vi "Solve1.vi"(8 "Error In":errorcluster, 11 "object in":refnum<class "2024_16.lvclass">) -> (0 "Error Out":errorcluster, 2 "Result":u64, 3 "object out":refnum<class "2024_16.lvclass">)   [LabVIEW 2023, in "2024_16.lvclass"]
uses:
  2024_16.lvclass
  2024_16.lvclass/2024_16.ctl
  Common/AOC_Direction.ctl
  Common/AOC_XY(I32).ctl
  Common/AOC_XY.ctl
panel:
  out "Array":T1(array[cluster])
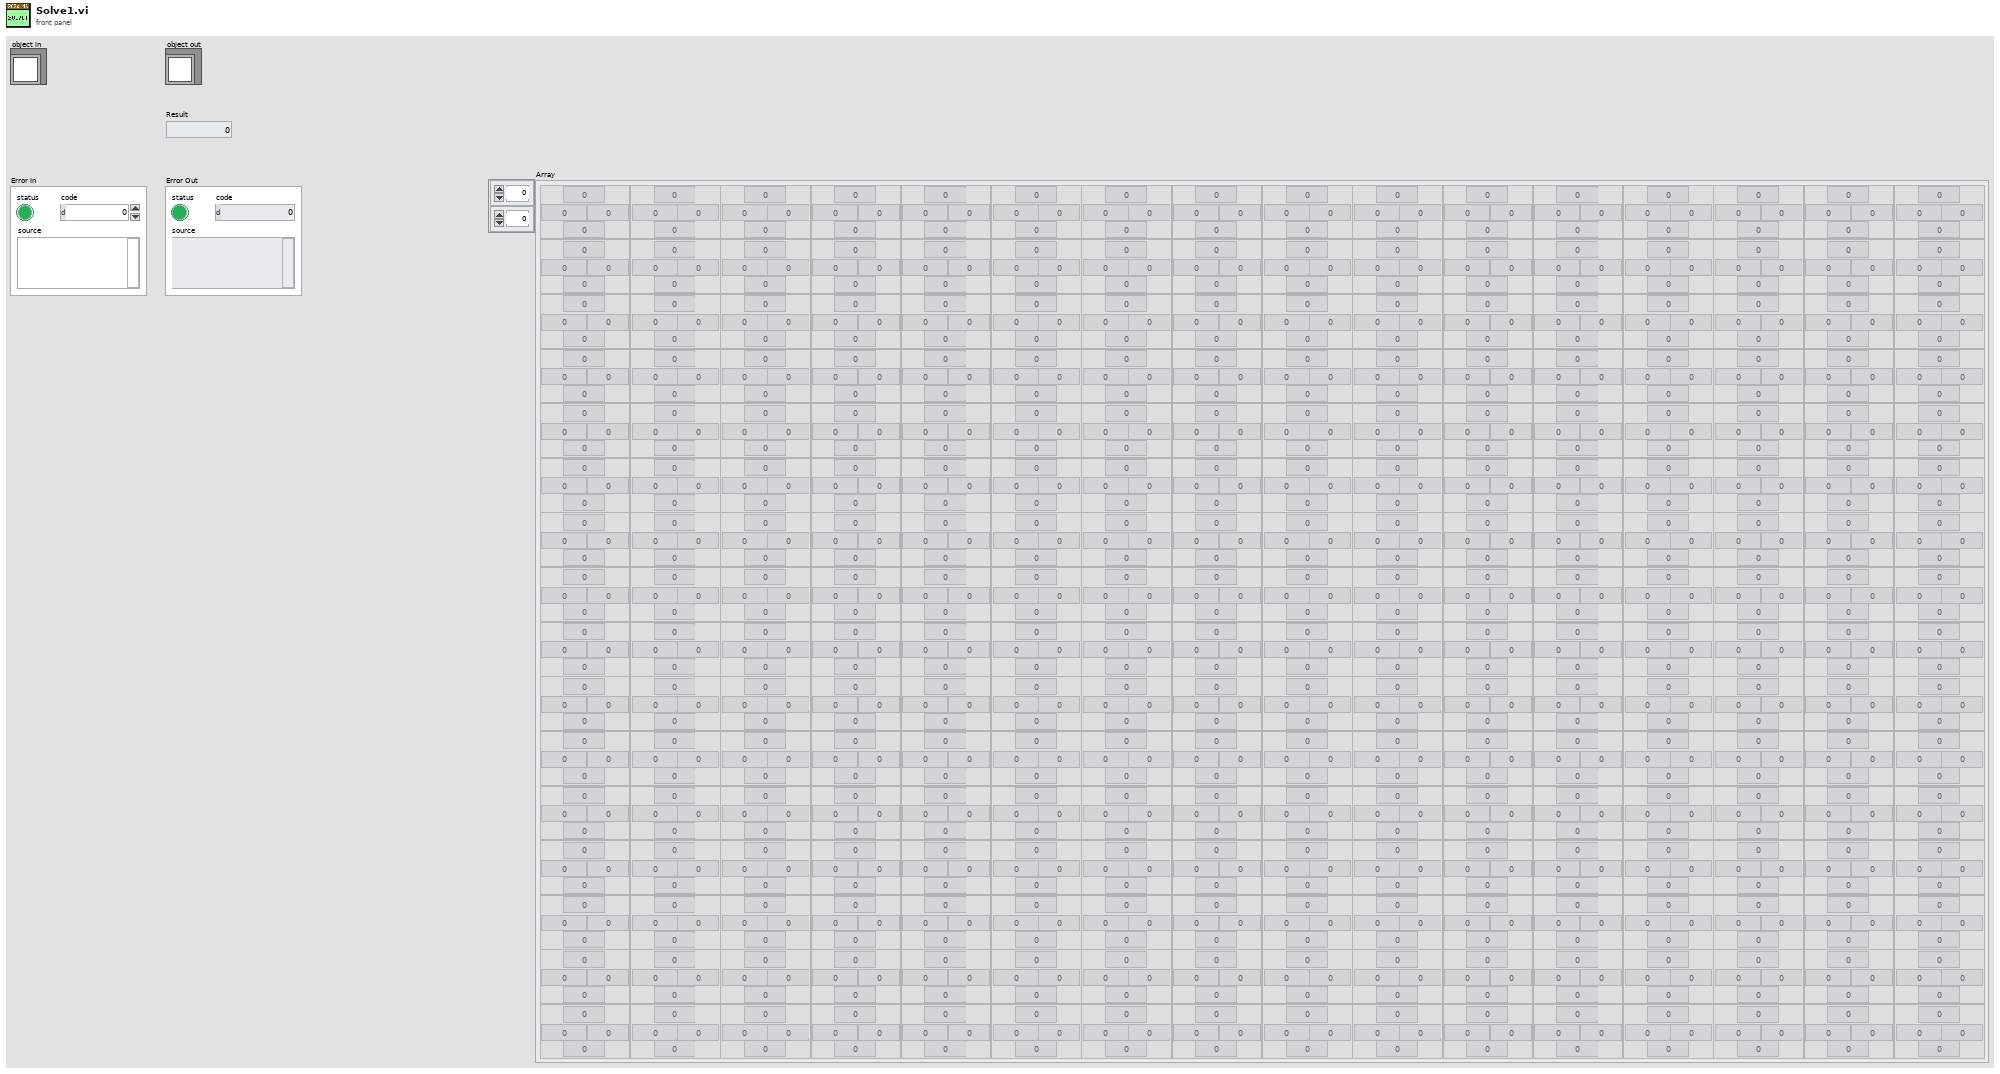
[diagram p1: front panel]
types:
  T1 = cluster{"Up":i32, "Right":i32, "Down":i32, "Left":i32}[][]
  T2 = cluster{"Up":u64, "Right":u64, "Down":u64, "Left":u64}
  T3 = typedef "AOC_Direction.ctl" = enum16{"Up", "Right", "Down", "Left"}
  T4 = typedef "AOC_XY(I32).ctl" = cluster{"X":i32, "Y":i32}
  T5 = map{T4, cluster{"Up":u64, "Right":u64, "Down":u64, "Left":u64}}
  T6 = typedef "AOC_XY.ctl" = cluster{"X":u64, "Y":u64}
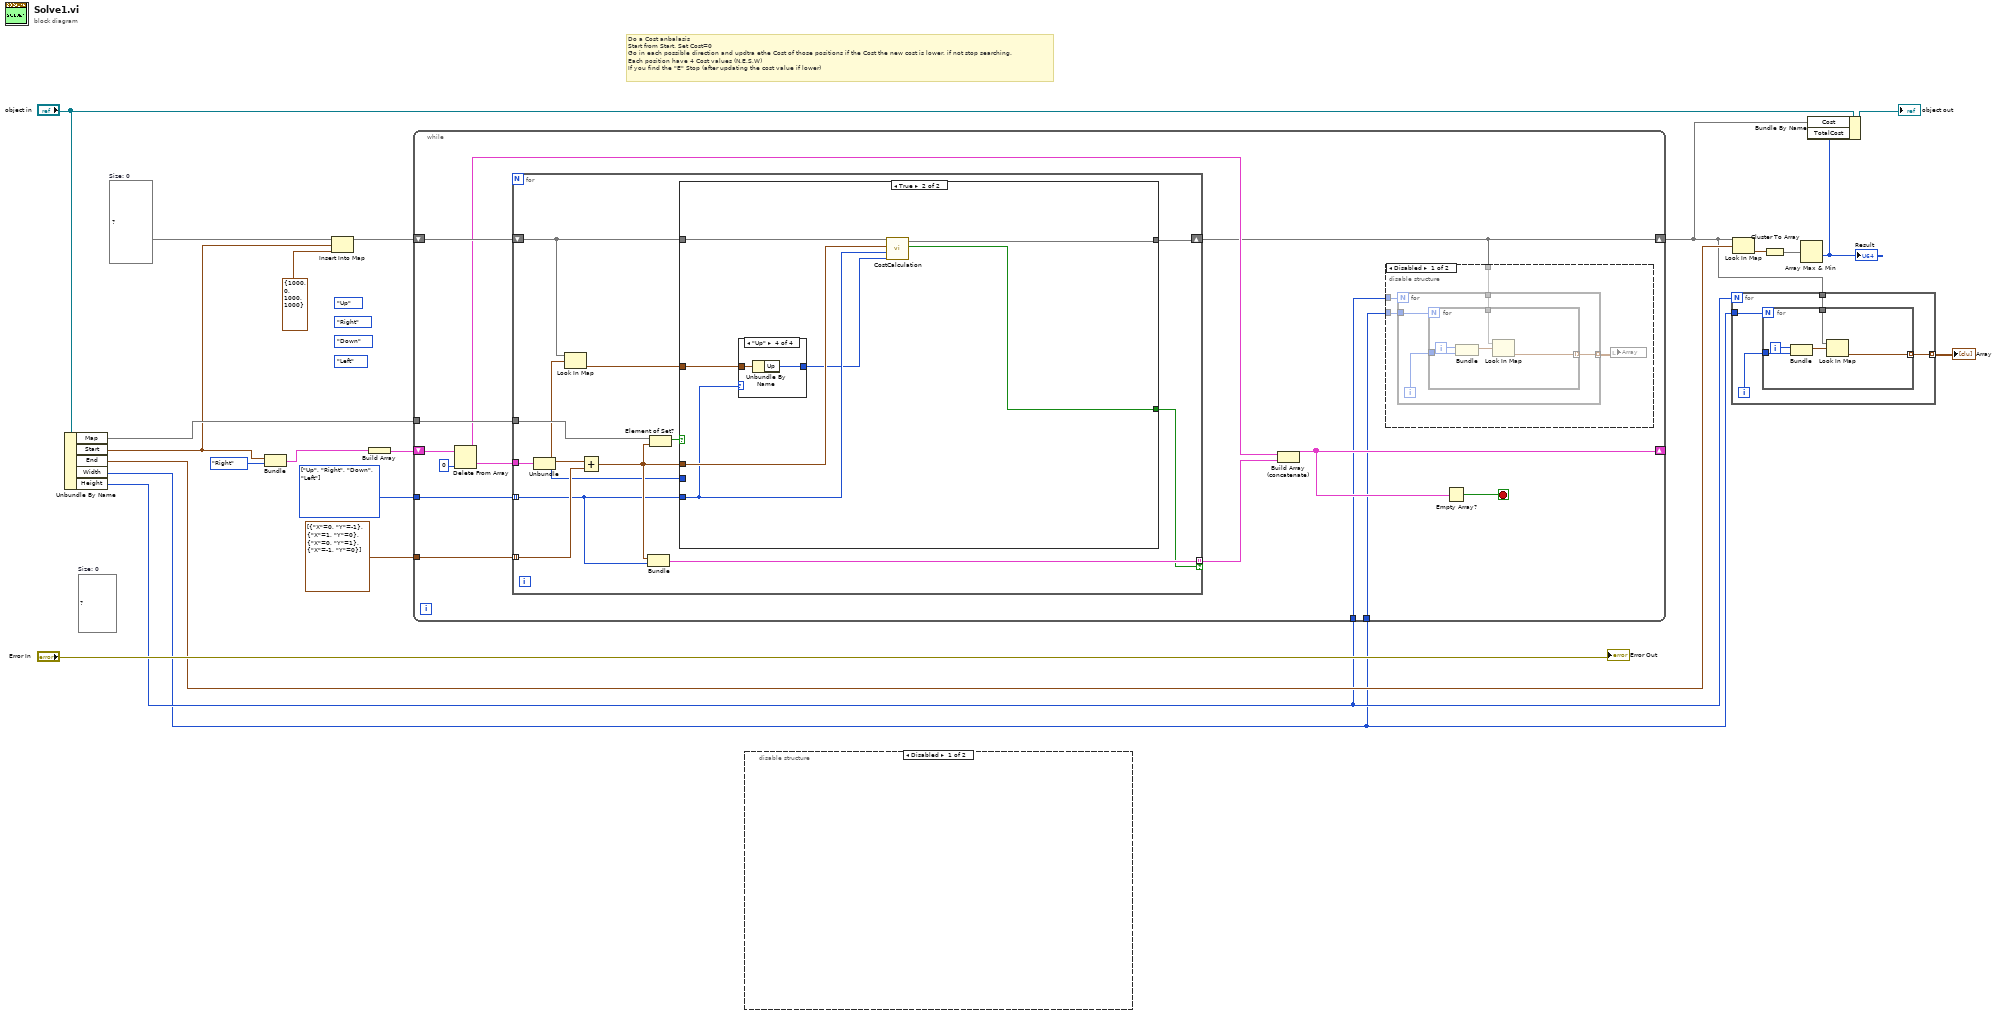
[diagram p0: block diagram]
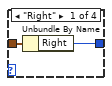
[diagram p5: hidden frame]
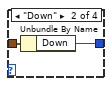
[diagram p6: hidden frame]
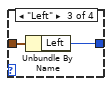
[diagram p7: hidden frame]
diagram:
  (unwired) AOC_Direction."Left" ("Enum")
  (unwired) AOC_Direction."Down" ("Enum")
  (unwired) AOC_Direction."Right" ("Enum")
  (unwired) AOC_Direction."Up" ("Enum")
  w16 = T3[] [enum."Up", enum."Right", enum."Down", enum."Left"] items=["Up", "Right", "Down", "Left"]
  w18 = T5 {}  # Size: 0
  (unwired) map{T6, i32} {}  # Size: 0
  # "Do a Cost anbalasis\nStart from Start. Set Cost=0\nGo in each possible direction and updtra ethe Cost of those positions if the Cost the new cost is lower, if not stop searching.\nEach position have 4 Cost values (N,E,S,W)\nIf you find the \"E\" Stop (after updating the cost value if lower)"
  n1 = Unbundle By Name("object in") -> ("Map"=w14:set{T4}, "Start"=w12:T4, "End"=w9:T4, "Width"=w2:i32, "Height"=w3:i32)
  n2 = Bundle("Start"=w12, AOC_Direction."Right") -> (w11:cluster{"Start":T4, T3})  [unwired: 1 in]
  n3 = Insert Into Map(map in=w18, key=w12, value=T2 {"Up"=1000, "Right"=0, "Down"=1000, "Left"=1000} ("input cluster")) -> (map out=w17:T5)  [unwired: 2 out]
  n4 = Build Array(w11) -> (w19:cluster{"Start":T4, T3}[])
  n5 = while {
    shift-right: [w26] -> _
    shift-left: w19 -> [w35]
    shift-right: [w23] -> w4
    shift-left: w17 -> [w30]
    tunnel: w16 -> [w33]
    tunnel: cluster{"X":i32, "Y":i32}[] [{"X"=0, "Y"=-1}, {"X"=1, "Y"=0}, {"X"=0, "Y"=1}, {"X"=-1, "Y"=0}] ("Array") -> [w32]
    tunnel: w14 -> [w31]
    tunnel: w2 -> [w25]
    tunnel: w3 -> [w24]
    stop <- w22 stop-if-true
    n6 = Delete From Array(array=w35, index=0) -> (deleted portion=w34:cluster{"Start":T4, T3}, array with subset deleted=w29:cluster{"Start":T4, T3}[])  [unwired: 1 in]
    n7 = for {
      tunnel: w34 -> [w59]
      tunnel: w33 -> [w50] mode=indexing
      tunnel: w32 -> [w61] mode=indexing
      tunnel: w31 -> [w60]
      shift-right: [w58] -> w23
      shift-left: w30 -> [w53]
      tunnel: [w54] -> w27 mode=indexing if=w49
      n8 = Unbundle(w59) -> ("Start"=w52:T4, w55:T3)
      n9 = Look In Map(map=w53, key=w52) -> (value=w51:T2)  [unwired: 1 in, 1 out]
      n10 = Add(x=w52, y=w61) -> (x+y=w56:T4)
      n11 = Bundle("Start"=w56, "Enum"=w50) -> (w54:cluster{"Start":T4, "Enum":T3})  [unwired: 1 in]
      n12 = Element of Set?(10:w56, 11:w60) -> (3:w57:bool)
      n13 = case shown="True" w57 {
        tunnel: w55 -> [_ _]
        tunnel: w50 -> [_ w64]
        tunnel: w53 -> [w62 w69]
        tunnel: [w62 w68] -> w58
        tunnel: w56 -> [_ w66]
        tunnel: w51 -> [_ w65]
        tunnel: [_ w67] -> w49
        frame False {
        }
        frame True {
          n14 = case shown="\"Up\"" w64 {
            tunnel: w65 -> [w71 w73 w75 w77]
            tunnel: [w70 w72 w74 w76] -> w63
            frame "Right" {
              n15 = Unbundle By Name(w71) -> ("Right"=w70:u64)
            }
            frame "Down" {
              n16 = Unbundle By Name(w73) -> ("Down"=w72:u64)
            }
            frame "Left" {
              n17 = Unbundle By Name(w75) -> ("Left"=w74:u64)
            }
            frame "Up" {
              n18 = Unbundle By Name(w77) -> ("Up"=w76:u64)
            }
          }
          n19 = call "CostCalculation.vi"("PrevisouCost"=w63, "Direction"=w64, "Position"=w66, "CostIn"=w69) -> ("CostLower"=w67:bool, "CostOut"=w68:T5)  [unwired: 4 in, 2 out]
        }
      }
    }
    n20 = Build Array (concatenate)(w29, w27) -> (w26:cluster{"Start":T4, "Enum":T3}[])
    n21 = disable-structure shown="Disabled" {
      disable-tunnel: w25 -> [w39 _]
      disable-tunnel: w24 -> [w38 _]
      disable-tunnel: w23 -> [w37 _]
      frame Disabled {
        n22 = for {
          N: w38 -> [_]
          tunnel: w39 -> [w43]
          tunnel: w37 -> [w41]
          tunnel: [w40] -> w36 mode=indexing
          i -> [w42]
          n23 = for {
            N: w43 -> [_]
            tunnel: w42 -> [w47]
            tunnel: w41 -> [w46]
            tunnel: [w44] -> w40 mode=indexing
            i -> [w48]
            n24 = Bundle(w48, w47) -> (w45:cluster{i32, i32})  [unwired: 1 in]
            n25 = Look In Map(map=w46, key=w45) -> (value=w44:T2)  [unwired: 1 in, 1 out]
          }
        }
        n26 = local write "Array"(w36) -> ()
      }
      frame Enabled {
      }
    }
    n27 = Empty Array?(array=w26) -> (empty?=w22:bool)
  }
  n28 = disable-structure shown="Disabled" {
    frame Disabled {
    }
    frame Enabled {
    }
  }
  n29 = for {
    N: w3 -> [_]
    tunnel: w2 -> [w81]
    tunnel: w4 -> [w79]
    tunnel: [w78] -> w1 mode=indexing
    i -> [w80]
    n30 = for {
      N: w81 -> [_]
      tunnel: w80 -> [w85]
      tunnel: w79 -> [w84]
      tunnel: [w82] -> w78 mode=indexing
      i -> [w86]
      n31 = Bundle(w86, w85) -> (w83:cluster{i32, i32})  [unwired: 1 in]
      n32 = Look In Map(map=w84, key=w83) -> (value=w82:T2)  [unwired: 1 in, 1 out]
    }
  }
  "Array" <- w1
  n33 = Look In Map(map=w4, key=w9) -> (value=w8:T2)  [unwired: 1 in, 1 out]
  n34 = Cluster To Array(cluster=w8) -> (array=w7:u64[])
  n35 = Array Max & Min(array=w7) -> (min value=w5:u64)  [unwired: 3 out]
  "Result" <- w5
  n36 = Bundle By Name(cluster="object in", "Cost"=w4, "TotalCost"=w5) -> (→"object out":refnum<class "2024_16.lvclass">)
  "Error Out" <- "Error In"
